vi "Read_LightIntensity.vi"(11 "LDR Input":tag) -> (3 "Boolean":bool)   [LabVIEW 2022 SP3]
uses:
  <vilib>/DAQmx/read.llb/DAQmx Read (Digital Bool 1Line 1Point).vi
  <vilib>/DAQmx/create/channels.llb/DAQmx Create Channel (DI-Digital Input).vi
  <vilib>/DAQmx/miscellaneous.llb/DAQmx Fill In Error Info.vi
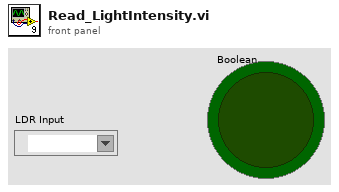
[diagram p1: front panel]
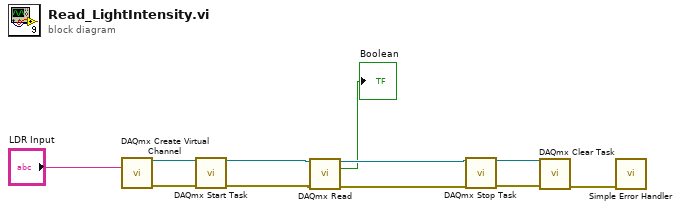
[diagram p0: block diagram]
diagram:
  n1 = call-poly <vilib>:"DAQmx Create Virtual Channel.vi"("lines"="LDR Input") -> ("task out"=w11:refnum<k21>, "error out"=w9:errorcluster)  [unwired: 13 in]
  n2 = call <vilib>:"DAQmx Start Task.vi"("task/channels in"=w11, "error in"=w9) -> ("task out"=w5:refnum<k21>, "error out"=w3:errorcluster)  [unwired: 12 in]
  n3 = call-poly <vilib>:"DAQmx Read.vi"("task/channels in"=w5, "error in"=w3) -> ("task out"=w4:refnum<k21>, "data"=→"Boolean":bool, "error out"=w2:errorcluster)  [unwired: 11 in]
  n4 = call <vilib>:"DAQmx Stop Task.vi"("task/channels in"=w4, "error in"=w2) -> ("task out"=w8:refnum<k21>, "error out"=w7:errorcluster)  [unwired: 12 in]
  n5 = call <vilib>:"DAQmx Clear Task.vi"("task in"=w8, "error in"=w7) -> ("error out"=w6:errorcluster)  [unwired: 13 in]
  n6 = call <vilib>:"Simple Error Handler.vi"("error in (no error)"=w6) -> ()  [unwired: 4 in, 5 out]
